vi "example test.vi"() -> ()   [LabVIEW 2014, in "Tagbus PID Module tests.lvlib"]
uses:
  Tagbus PID Module tests.lvlib
  module/configuration/PID Module configuration.lvclass
  module/execution/PID Module runtime.lvclass
  editor node/PID array element.ctl
  module/configuration/PID Loop/String Parameters.ctl
  <vilib>/NI/Tag Bus/tag/Data Type.ctl
  <vilib>/NI/Tag Bus/tag/tag descriptor.lvclass
  <vilib>/NI/Tag Bus/dictionary/data dictionary.lvclass/data dictionary.ctl
  <vilib>/NI/Tag Bus/dictionary/lookup polymorphs/locate double.vi
  <vilib>/NI/Tag Bus/table/data polymorphs/write one/write Double.vi
  <vilib>/NI/Tag Bus/table/data polymorphs/read one/read Double.vi
  <vilib>/NI/Tag Bus/dictionary/search/find data index.vi
  <vilib>/NI/Tag Bus/dictionary/search/search string list.vi
  <vilib>/NI/Tag Bus/dictionary/tag not found.vi
  <vilib>/NI/Tag Bus/dictionary/data dictionary.lvclass
  <vilib>/NI/Tag Bus/table/data table.lvlib
  <vilib>/NI/Configuration Framework/serializable configuration/NISE_CEF_serializable configuration.lvclass
  editor node/PID Module editor node.lvclass
  module/configuration/PID Loop.lvclass
panel:
  out "final error":errorcluster
  out "output error":errorcluster
  out "input error":errorcluster
  out "output lookup error":errorcluster
  out "no data written":bool
  out "input lookup error":errorcluster
  out "init error":errorcluster
  out "correct execution settings":bool
  out "serialization problem":errorcluster
  out "invalid configuration":errorcluster
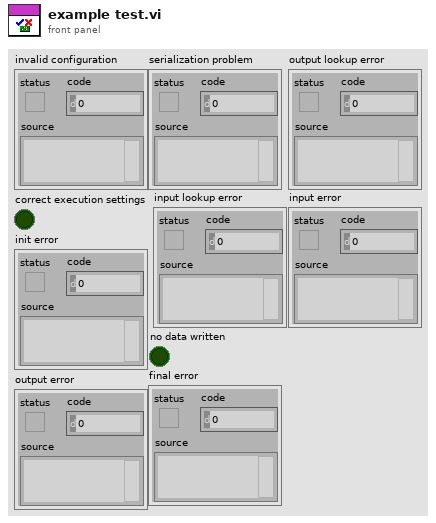
[diagram p1: front panel]
types:
  T1 = typedef "PID Loop.lvclass/String Parameters.ctl" = enum16{"Setpoint", "Process Variable", "Output", "Proportional Gain", "Integral Time", "Derivative Time", "Range High", "Range Low"}
  T2 = typedef "PID Module editor node.lvclass/PID array element.ctl" = cluster{"Loop ID":string, "Tags":cluster{"Setpoint":string, "Process Variable":string, "Output":string}, "Gains":cluster{"P":dbl, "I":dbl, "D":dbl}, "Range":cluster{"High":dbl, "Low":dbl}}
  T3 = typedef "tag bus.lvlib/tag descriptor.lvclass/Data Type.ctl" = enum16{"Double", "Single", "I64", "I32", "I16", "I8", "U64", "U32", "U16", "U8", "Boolean", "String", "Array of Double", "Array of Single", "Array of I64", "Array of I32", "Array of I16", "Array of I8", "Array of U64", "Array of U32", "Array of U16", "Array of U8", "Array of Boolean", "Array of String"}
  T4 = typedef "TBM channel.lvclass/data tables.ctl" = cluster{"input data":T5, "processing parameter":T5, "processing result":T5, "output data":T5}
  T5 = typedef "tag bus.lvlib/dictionary table pair.ctl" = cluster{"data dictionary":refnum<class "data dictionary.lvclass">, "data table":T6}
  T6 = typedef "tag bus.lvlib/data table.lvlib/data table.ctl" = cluster{"Double":dbl[], "Single":sgl[], "I64":i64[], "I32":i32[], "I16":i16[], "I8":i8[], "U64":u64[], "U32":u32[], "U16":u16[], "U8":u8[], "Boolean":bool[], "String":string[], "Array of Double":cluster{"DBL Array":dbl[]}[], "Array of Single":cluster{"SGL Array":sgl[]}[], "Array of I64":cluster{"I64 Array":i64[]}[], "Array of I32":cluster{"I32 Array":i32[]}[], "Array of I16":cluster{"I16 Array":i16[]}[], "Array of I8":cluster{"I8 Array":i8[]}[], "Array of U64":cluster{"U64 Array":u64[]}[], "Array of U32":cluster{"U32 Array":u32[]}[], "Array of U16":cluster{"U16 Array":u16[]}[], "Array of U8":cluster{"U8 Array":u8[]}[], "Array of Boolean":cluster{"Boolean Array":bool[]}[], "Array of String":cluster{"String Array":string[]}[]}
  T7 = typedef "TBM module execution interface.lvclass/execution settings.ctl" = cluster{"reads inputs":bool, "processes data":bool, "writes outputs":bool}
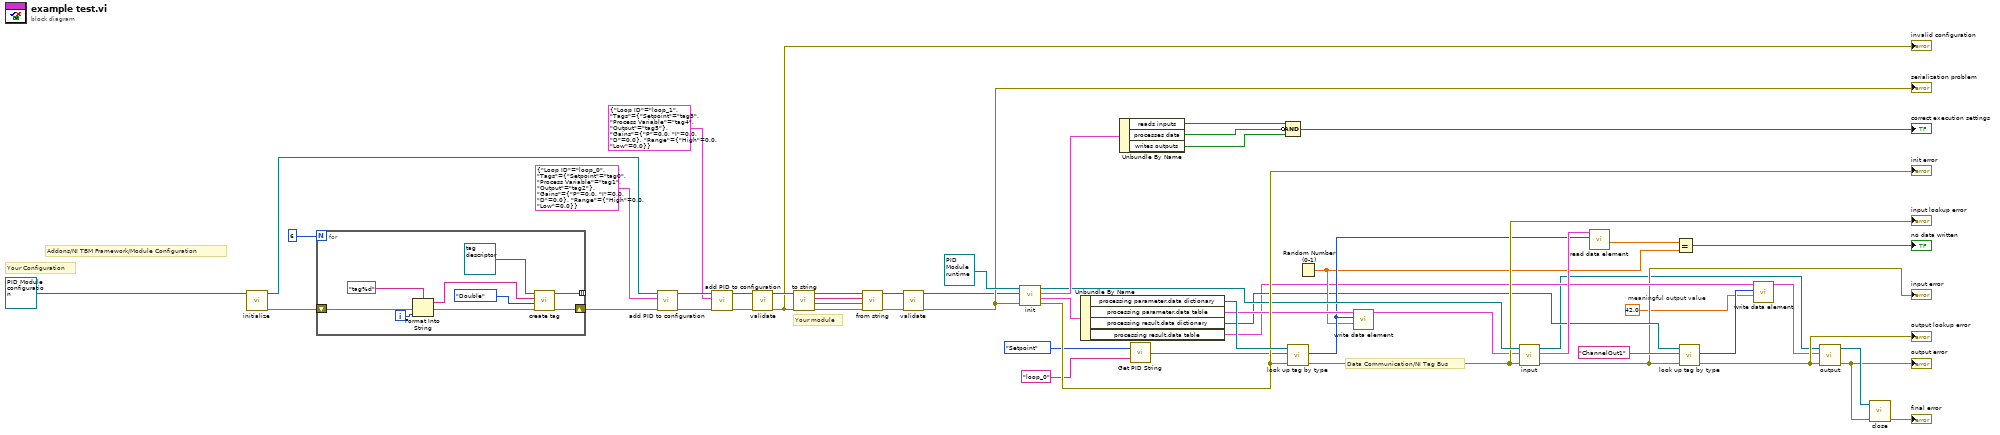
[diagram p0: block diagram]
diagram:
  w21 = 42.0  # meaningful output value
  # "Data Communication/NI Tag Bus"
  # "Your module"
  # "Your Configuration"
  # "Addons/NI TBM Framework/Module Configuration"
  n1 = call <vilib>:"initialize.vi"("configuration in"=refnum<class "PID Module configuration.lvclass"> refnum ("tag bus configurable plugin module configuration")) -> ("error out"=w2:errorcluster, "configuration out"=w10:refnum<class "PID Module configuration.lvclass">)  [unwired: 8 in, 1 out]
  n2 = for {
    N: 6 -> [_]
    tunnel: [w60] -> _ mode=indexing
    shift-right: [w55] -> w1
    shift-left: w2 -> [w56]
    i -> [w63]
    n3 = Format Into String(format string="tag%d", error in=w56, w63) -> (resulting string=w59:string, error out=w57:errorcluster)  [unwired: 1 in]
    n4 = call-dynamic "create tag.vi"("error in"=w57, "data type"=Data_Type."Double", "name"=w59, "tag descriptor in"=refnum<class "tag descriptor.lvclass"> refnum) -> ("error out"=w55:errorcluster, "tag descriptor out"=w60:refnum<class "tag descriptor.lvclass">)  [unwired: 6 in]
  }
  n5 = call "add PID to configuration.vi"("error in"=w1, "PID Element in"=T2 {"Loop ID"="loop_0", "Tags"={"Setpoint"="tag0", "Process Variable"="tag1", "Output"="tag2"}, "Gains"={"P"=0.0, "I"=0.0, "D"=0.0}, "Range"={"High"=0.0, "Low"=0.0}}, "Tagbus PID Module configuration in"=w10) -> ("error out"=w11:errorcluster, "Tagbus PID Module configuration out"=w13:refnum<class "PID Module configuration.lvclass">)  [unwired: 7 in]
  n6 = call "add PID to configuration.vi"("error in"=w11, "PID Element in"=T2 {"Loop ID"="loop_1", "Tags"={"Setpoint"="tag3", "Process Variable"="tag4", "Output"="tag5"}, "Gains"={"P"=0.0, "I"=0.0, "D"=0.0}, "Range"={"High"=0.0, "Low"=0.0}}, "Tagbus PID Module configuration in"=w13) -> ("error out"=w9:errorcluster, "Tagbus PID Module configuration out"=w12:refnum<class "PID Module configuration.lvclass">)  [unwired: 7 in]
  n7 = call-dynamic "validate.vi"("error in"=w9, "Tagbus PID Module configuration in"=w12) -> ("error out"=w53:errorcluster, "Tagbus PID Module configuration out"=w54:refnum<class "PID Module configuration.lvclass">)  [unwired: 8 in]
  "invalid configuration" <- w53
  n8 = call-dynamic "to string.vi"("error in"=w53, "Tagbus PID Module configuration in"=w54) -> ("error out"=w49:errorcluster, "data"=w50:string, "version"=w51:string, "Tagbus PID Module configuration out"=w52:refnum<class "PID Module configuration.lvclass">)  [unwired: 6 in]
  n9 = call-dynamic "from string.vi"("error in"=w49, "data"=w50, "version"=w51, "Tagbus PID Module configuration in"=w52) -> ("error out"=w47:errorcluster, "Tagbus PID Module configuration out"=w48:refnum<class "PID Module configuration.lvclass">)  [unwired: 6 in]
  n10 = call-dynamic "validate.vi"("error in"=w47, "Tagbus PID Module configuration in"=w48) -> ("error out"=w45:errorcluster, "Tagbus PID Module configuration out"=w44:refnum<class "PID Module configuration.lvclass">)  [unwired: 8 in]
  "serialization problem" <- w45
  n11 = call-dynamic "init.vi"("error in"=w45, "TBM module configuration in"=w44, "Tagbus PID Module runtime in"=refnum<class "PID Module runtime.lvclass"> refnum ("tag bus configurable plugin module")) -> ("error out"=w36:errorcluster, "data allocations"=w38:T4, "execution settings"=w43:T7, "Tagbus PID Module runtime out"=w34:refnum<class "PID Module runtime.lvclass">)  [unwired: 5 in]
  "init error" <- w36
  n12 = Unbundle By Name(w38) -> ("processing parameter.data dictionary"=w37:refnum<class "data dictionary.lvclass">, "processing parameter.data table"=w35:T6, "processing result.data dictionary"=w26:refnum<class "data dictionary.lvclass">, "processing result.data table"=w23:T6)
  n13 = Unbundle By Name(w43) -> ("reads inputs"=w40:bool, "processes data"=w42:bool, "writes outputs"=w41:bool)
  n14 = call "Get PID String.vi"("PID Loop ID"="loop_0", "PID Parameter"=String_Parameters."Setpoint") -> ("Parameter String"=w4:string)
  n15 = Compound Arithmetic op=AND(w40, invert w42, w41) -> (→"correct execution settings":bool)
  n16 = call-poly <vilib>:"look up tag by type.vi"("error in"=w36, "name"=w4, "data dictionary in"=w37) -> ("error out"=w33:errorcluster, "index"=w30:i32)  [unwired: 6 in, 1 out]
  "input lookup error" <- w33
  n17 = Random Number (0-1)() -> (number: 0 to 1=w29:dbl)
  n18 = call-poly <vilib>:"write data element.vi"("value"=w29, "index"=w30, "data table in"=w35) -> ("data table out"=w32:T6)  [unwired: 8 in]
  n19 = call-dynamic "input.vi"("error in"=w33, "input allocation"=w32, "module in"=w34) -> ("error out"=w22:errorcluster, "input data"=w31:T6, "module out"=w19:refnum<class "PID Module runtime.lvclass">)  [unwired: 6 in]
  "input error" <- w22
  n20 = call-poly <vilib>:"read data element.vi"("index"=w30, "data table in"=w31) -> ("value"=w28:dbl)  [unwired: 8 in, 1 out]
  n21 = Equal?(x=w28, y=w29) -> (x = y?=→"no data written":bool)
  n22 = call-poly <vilib>:"look up tag by type.vi"("error in"=w22, "name"="ChannelOut1" ("channel name"), "data dictionary in"=w26) -> ("error out"=w20:errorcluster, "index"=w24:i32)  [unwired: 6 in, 1 out]
  "output lookup error" <- w20
  n23 = call-poly <vilib>:"write data element.vi"("value"=w21, "index"=w24, "data table in"=w23) -> ("data table out"=w18:T6)  [unwired: 8 in]
  n24 = call-dynamic "output.vi"("error in"=w20, "output data"=w18, "module in"=w19) -> ("error out"=w16:errorcluster, "module out"=w17:refnum<class "PID Module runtime.lvclass">)  [unwired: 6 in, 1 out]
  "output error" <- w16
  n25 = call-dynamic "close.vi"("error in"=w16, "Tagbus PID Module runtime in"=w17) -> ("error out"=→"final error":errorcluster)  [unwired: 9 in]
